vi "AutoMove.vi"(6 "Wait":u32=500, 8 "Right Power":i8=100, 9 "Left Power":i8=100, 11 "BrickReference in":T1) -> (3 "BrickReference out":T1)   [LabVIEW 2012, in "BlockParty4150.lvrbt"]
uses:
  BlockParty4150.lvrbt
  <vilib>/NXT/Subs/LVHSConnector.ctl
  <vilib>/NXT/LegoClasses/BrickReference/BrickReference.lvclass
  <vilib>/NXT/Hardware/Plugins/Tetrix DC Motor/TetrixDCMotorAddress.ctl
  <vilib>/NXT/NXTIO Xnodes/NXTIONodeSubVIs/TETRIX IO Move DC Motors.vi
  <vilib>/NXT/NXTIO Xnodes/NXTIONodeSubVIs/TETRIX IO Stop DC Motors.vi
  <vilib>/NXT/NXTIO Xnodes/AddressXNode/NXTIOAddress.xnode
  <vilib>/NXT/NXTIO Xnodes/NXTIOXNode/NXTIO.xnode
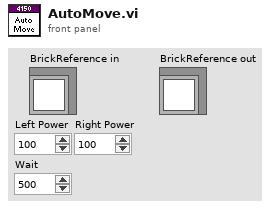
[diagram p1: front panel]
types:
  T1 = typedef "LVHSConnector.ctl" = refnum<class "BrickReference.lvclass">
  T2 = typedef "TetrixDCMotorAddress.ctl" = i16
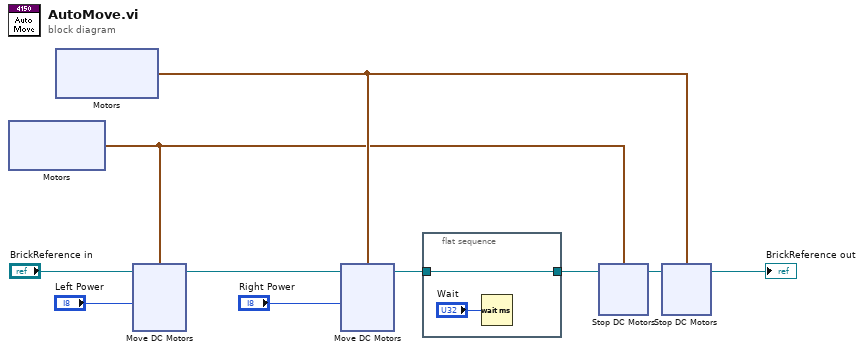
[diagram p0: block diagram]
diagram:
  n1 = xnode "Motors"() -> ("Motor"=w1:cluster{"TetrixDCMotor":T2, "TetrixDCMotor":T2})
  n2 = xnode "Motors"() -> ("Motor"=w2:cluster{"TetrixDCMotor":T2, "TetrixDCMotor":T2})
  n3 = xnode "Move DC Motors"("Power/Speed 2"="Left Power", "Power/Speed 1"="Left Power", "Motors"=w1, "NXT"="BrickReference in") -> ("NXT"=w6:T1)
  n4 = xnode "Move DC Motors"("Power/Speed 2"="Right Power", "Power/Speed 1"="Right Power", "Motors"=w2, "NXT"=w6) -> ("NXT"=w9:T1)
  n5 = flat-sequence {
    tunnel: [w11] -> w7
    tunnel: w9 -> [w11]
    frame #0 {
      n6 = Wait (ms)(milliseconds to wait="Wait") -> ()  [unwired: 1 out]
    }
  }
  n7 = xnode "Stop DC Motors"("Motors"=w1, "NXT"=w7) -> ("NXT"=w8:T1)
  n8 = xnode "Stop DC Motors"("Motors"=w2, "NXT"=w8) -> ("NXT"=→"BrickReference out":T1)
